vi "5_shift_register_application.vi"() -> ()   [LabVIEW 2017]
panel:
  out "Waveform Chart":cluster{dbl, "Celsius":dbl}(graph)
  in  "stop":bool
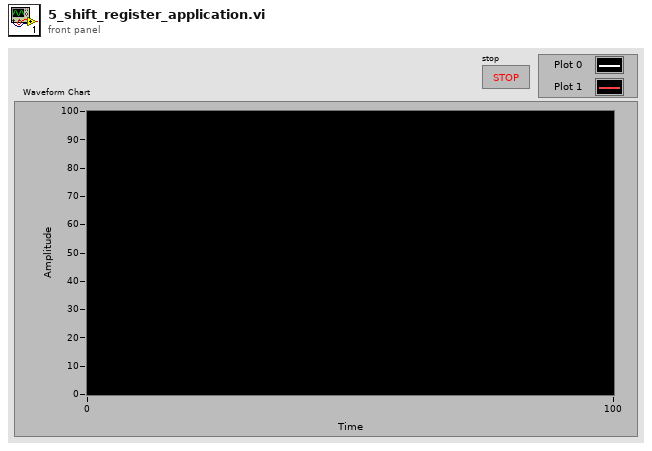
[diagram p1: front panel]
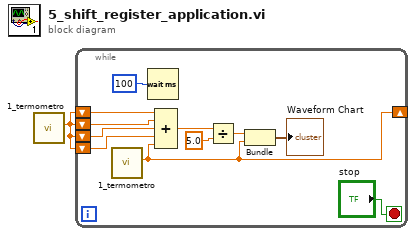
[diagram p0: block diagram]
diagram:
  n1 = call "1_termometro.vi"() -> ("Celsius"=w1:dbl)  [unwired: 1 in, 3 out]
  n2 = while {
    shift-right: [w2] -> _
    shift-left: w1 -> [w10]
    shift-left: w1 -> [w8]
    shift-left: w1 -> [w9]
    shift-left: w1 -> [w7]
    stop <- "stop" stop-if-true
    n3 = call "1_termometro.vi"() -> ("Celsius"=w2:dbl)  [unwired: 1 in, 3 out]
    n4 = Wait (ms)(milliseconds to wait=u32 100) -> ()  [unwired: 1 out]
    n5 = Compound Arithmetic op=ADD(w10, w9, w8, w7, w2) -> (w6:dbl)
    n6 = Divide(x=w6, y=5.0) -> (x/y=w3:dbl)
    n7 = Bundle(w3, "Celsius"=w2) -> (→"Waveform Chart":cluster{dbl, "Celsius":dbl})  [unwired: 1 in]
  }
